vi "LcWebView_AlertDialog_Custom Right-to-left support for Arabic, Persian, Hebrew, and other RTL languages.vi"() -> ()   [LabVIEW 2018, in "LcWebView.lvclass"]
uses:
  LcWebView.lvclass
  C:/Users/ziggz/OneDrive/Documents/GitHub/LcWebView2/LcWebView/LcWebView_class/data/Microsoft.Web.WebView2.WinForms.dll
  data/Microsoft.Web.WebView2.WinForms.dll
panel:
  out "BrowserProcessId":u32
  in  "stop":bool
  out "Result":string
  out "Status Message":string
  in  "Web":refnum<k24>(container)
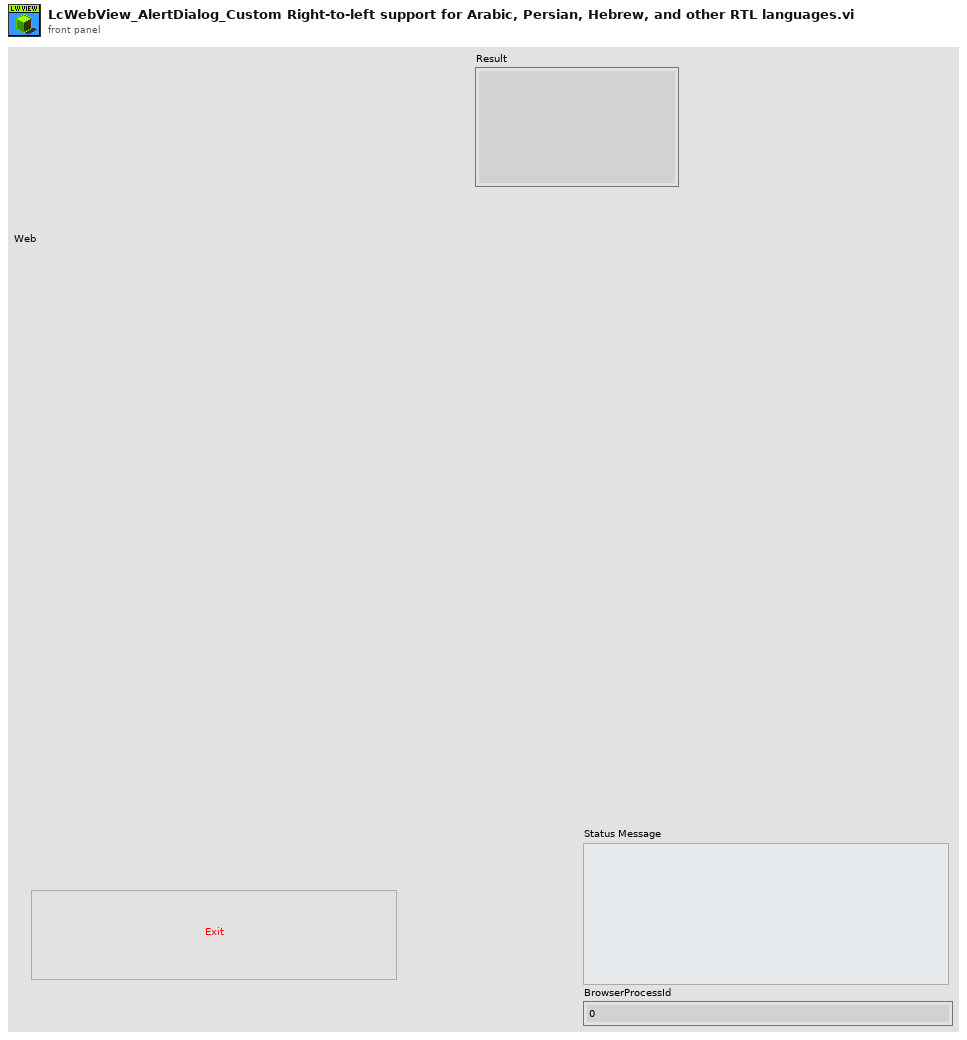
[diagram p1: front panel]
types:
  T1 = cluster{"title":string, "html":string, "timer":dbl, "timerProgressBar":bool, "didOpen":string, "willClose":string}
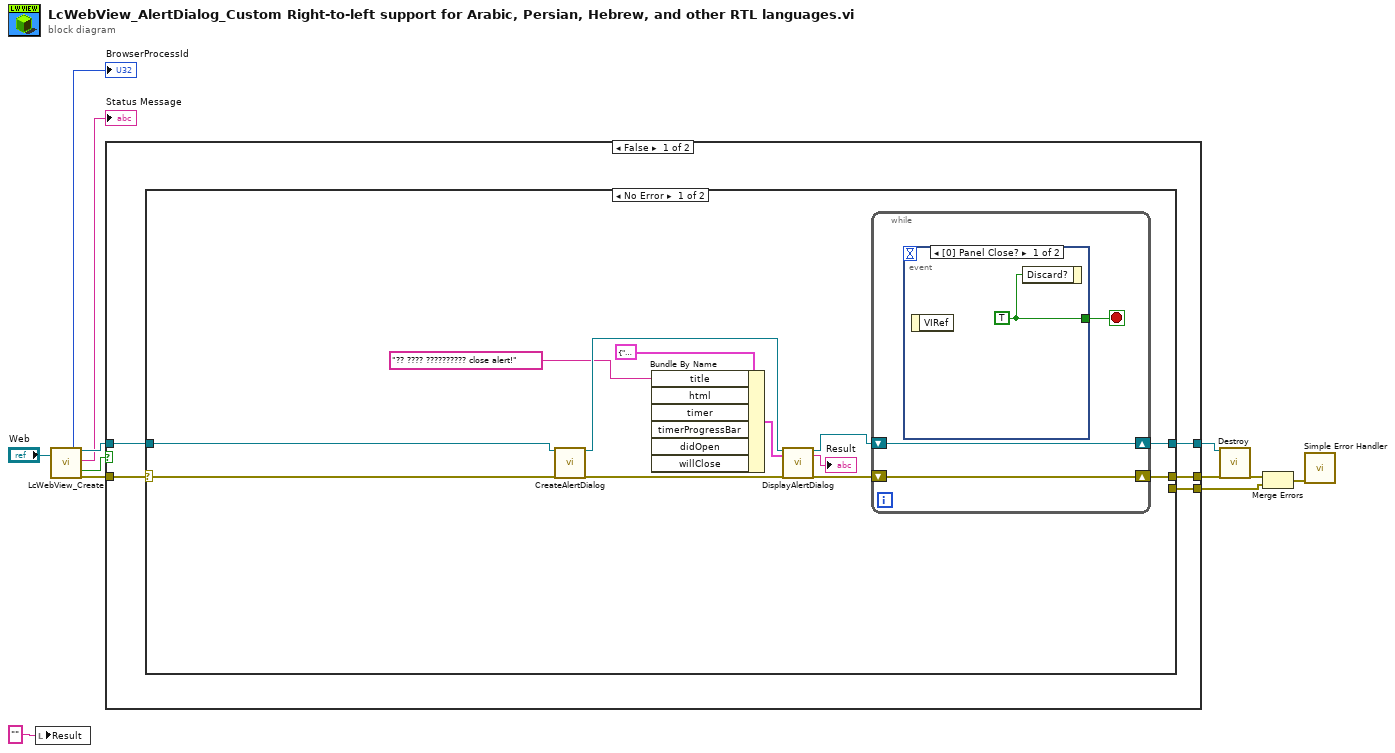
[diagram p0: block diagram]
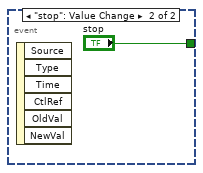
[diagram p2: hidden frame]
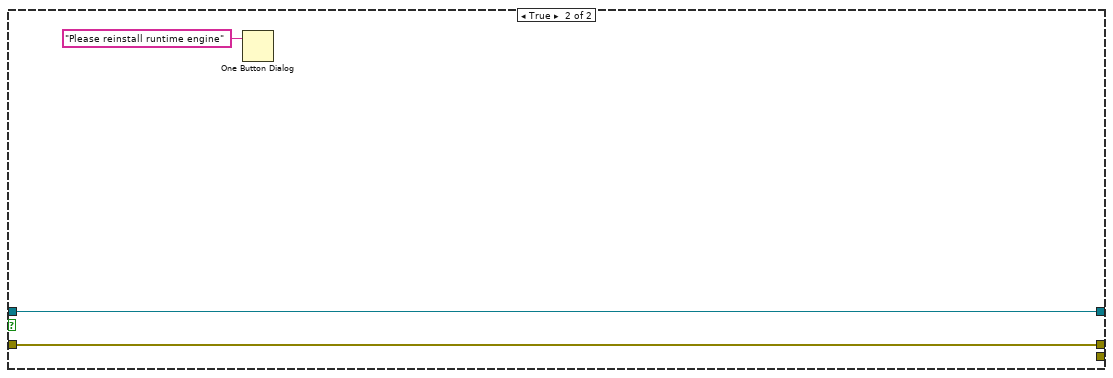
[diagram p4: hidden frame]
diagram:
  n1 = local write "Result"("" ("Result")) -> ()
  n2 = call "LcWebView_Create.vi"("Webview container"="Web") -> ("BrowserProcessId"=→"BrowserProcessId":u32, "reference out"=w11:refnum<class "LcWebView.lvclass">, "Status Message"=→"Status Message":string, "Reinstall Runtime"=w4:bool, "Error Out"=w10:errorcluster)  [unwired: 11 in, 3 out]
  n3 = case shown="False" w4 {
    tunnel: w11 -> [w17 w39]
    tunnel: w10 -> [w16 w38]
    tunnel: [w15 w39] -> w9
    tunnel: [w13 w38] -> w8
    tunnel: [w14 _] -> w5
    frame False {
      n4 = case shown="No Error" w16 {
        selector: w16 -> [w26 w35]
        tunnel: w17 -> [w27 w36]
        tunnel: [w28 w36] -> w15
        tunnel: [w29 _] -> w13
        tunnel: [_ w35] -> w14
        frame No Error {
          n5 = call-dynamic "CreateAlertDialog.vi"("reference in"=w27, "Error In"=w26) -> ("reference out"=w25:refnum<class "LcWebView.lvclass">, "Error Out"=w24:errorcluster)  [unwired: 16 in]
          n6 = Bundle By Name(cluster=T1 {"title"="", "html"="", "timer"=0.0, "timerProgressBar"=TRUE, "didOpen"="", "willClose"=""}, "title"="?? ???? ?????????? close alert!") -> (w21:T1)  [unwired: 5 in]
          n7 = call-dynamic "DisplayAlertDialog.vi"("reference in"=w25, "Message"=w21, "Error In"=w24) -> ("reference out"=w23:refnum<class "LcWebView.lvclass">, "Result"=→"Result":string, "Error Out"=w22:errorcluster)  [unwired: 14 in]
          n8 = while {
            shift-right: [w32] -> w28
            shift-left: w23 -> [w32]
            shift-right: [w31] -> w29
            shift-left: w22 -> [w31]
            stop <- w30 stop-if-true
            n9 = event shown="[0] Panel Close?" {
              selector: _ -> [_ _]
              dyn-events: _ -> [_ _]
              timeout: _ -> [_ _]
              tunnel: [w33 "stop"] -> w30
              event Panel Close? {
                w33 = TRUE ("Discard?")
                n10 = event-data() -> ()  [unwired: 1 in, 1 out]
                n11 = event-data("Discard?"=w33) -> ()  [unwired: 1 in, 1 out]
              }
              event "stop": Value Change {
                n12 = event-data() -> ()  [unwired: 1 in, 6 out]
              }
            }
          }
        }
        frame Error {
        }
      }
    }
    frame True {
      n13 = One Button Dialog(message="Please reinstall runtime engine") -> ()  [unwired: 1 in, 1 out]
    }
  }
  n14 = call-dynamic "Destroy.vi"("reference in"=w9, "Error In"=w8) -> ("Error Out"=w7:errorcluster)  [unwired: 16 in, 1 out]
  n15 = Merge Errors(w7, w5) -> (w2:errorcluster)
  n16 = call <vilib>:"Simple Error Handler.vi"("error in (no error)"=w2) -> ()  [unwired: 4 in, 5 out]
